vi "GetAllControlReferences.vi"(8 "error in (no error)":errorcluster, 10 "list tab?":bool=TRUE, 11 "VI Refnum in":refnum<vi>) -> (0 "error out":errorcluster, 2 "Ctrl Refs out":refnum<vi>[](array[refnum]), 3 "VI Refnum out":refnum<vi>)   [LabVIEW 2017]
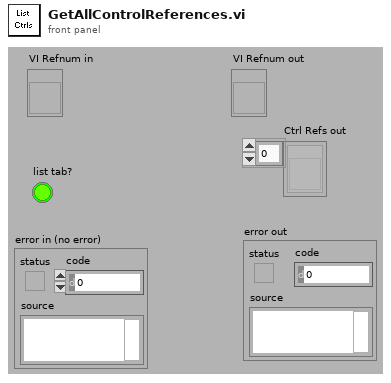
[diagram p1: front panel]
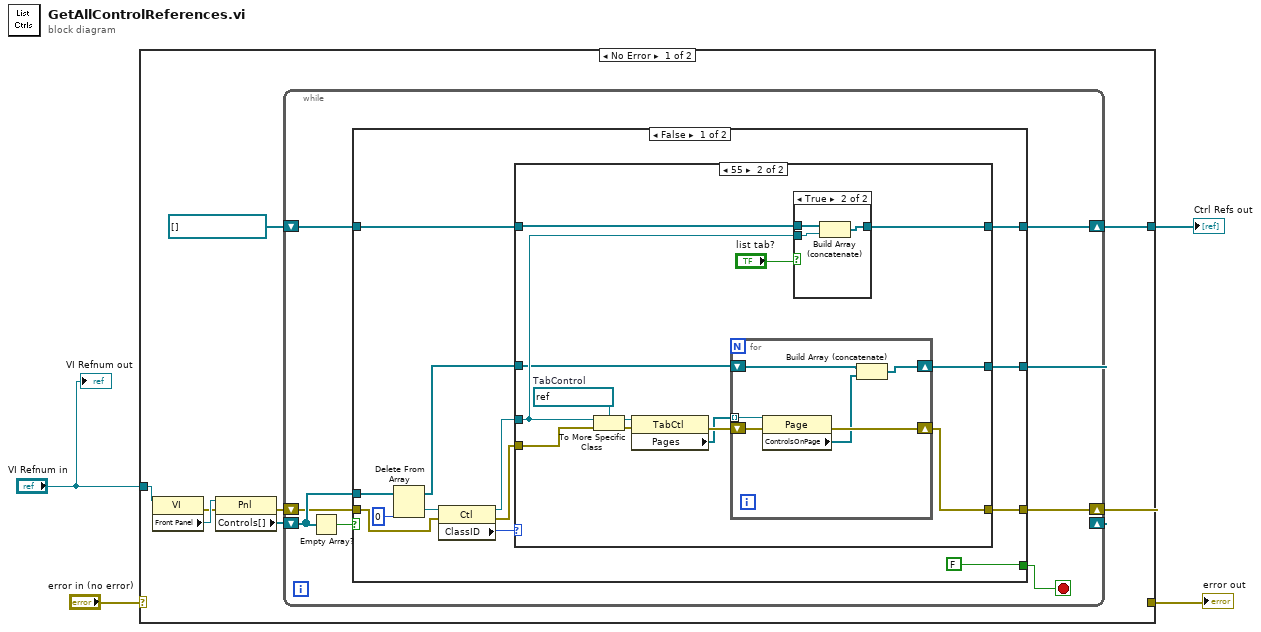
[diagram p0: block diagram]
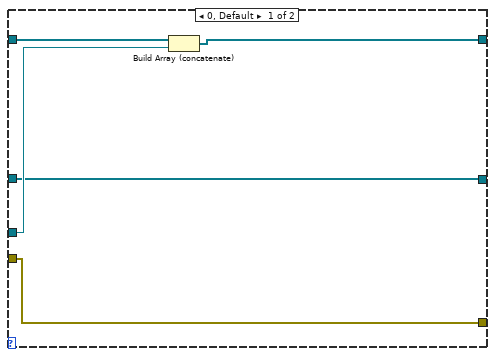
[diagram p2: hidden frame]
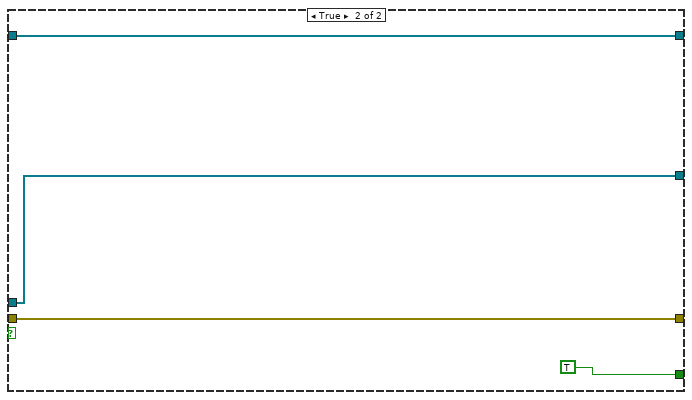
[diagram p4: hidden frame]
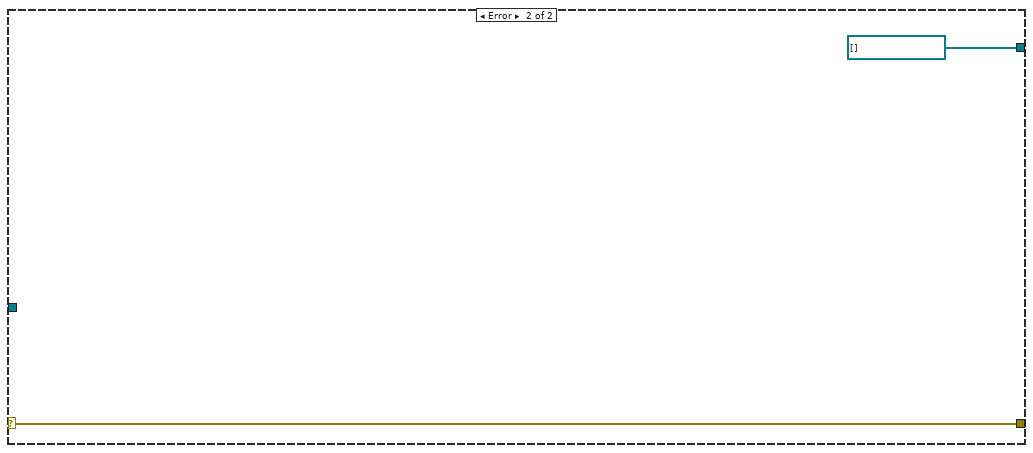
[diagram p5: hidden frame]
diagram:
  n1 = case shown="No Error" "error in (no error)" {
    selector: "error in (no error)" -> [_ w67]
    tunnel: [w6 w67] -> w3
    tunnel: "VI Refnum in" -> [w5 _]
    tunnel: [w8 refnum<vi>[] []] -> w1
    frame No Error {
      n2 = property class="VI"(reference=w5) -> (error out=w11:errorcluster, "Front Panel"=w12:refnum<vi>)  [unwired: 1 in, 1 out]
      n3 = property class="Pnl"(reference=w12, error in=w11) -> (error out=w9:errorcluster, "Controls[]"=w10:refnum<vi>[])  [unwired: 1 out]
      n4 = while {
        shift-right: [w17] -> _
        shift-left: w10 -> [w18]
        shift-right: [w13] -> w6
        shift-left: w9 -> [w16]
        shift-right: [w14] -> w8
        shift-left: refnum<vi>[] [] -> [w15]
        stop <- w19 stop-if-true
        n5 = Empty Array?(array=w18) -> (empty?=w20:bool)
        n6 = case shown="False" w20 {
          tunnel: [FALSE TRUE] -> w19
          tunnel: w18 -> [w31 w65]
          tunnel: [w21 w65] -> w17
          tunnel: w16 -> [w29 w62]
          tunnel: w15 -> [w26 w64]
          tunnel: [w25 w64] -> w14
          tunnel: [w23 w62] -> w13
          frame False {
            n7 = Delete From Array(array=w31, index=0) -> (deleted portion=w30:refnum<vi>, array with subset deleted=w22:refnum<vi>[])  [unwired: 1 in]
            n8 = property class="Ctl"(reference=w30, error in=w29) -> (reference out=w27:refnum<vi>, error out=w24:errorcluster, "ClassID"=w28:u32)
            n9 = case shown="55" w28 {
              tunnel: w27 -> [w37 w43]
              tunnel: w26 -> [w38 w44]
              tunnel: [w36 w41] -> w25
              tunnel: w24 -> [w35 w46]
              tunnel: [w35 w42] -> w23
              tunnel: w22 -> [w34 w40]
              tunnel: [w34 w39] -> w21
              frame 0, Default {
                n10 = Build Array (concatenate)(w38, w37) -> (w36:refnum<vi>[])
              }
              frame 55 {
                w47 = refnum<vi> refnum  # TabControl
                n11 = To More Specific Class(target class=w47, reference=w43, error in=w46) -> (specific class reference=w48:refnum<vi>, error out=w49:errorcluster)
                n12 = property class="TabCtl"(reference=w48, error in=w49) -> (error out=w51:errorcluster, "Pages"=w50:refnum<vi>[])  [unwired: 1 out]
                n13 = for {
                  tunnel: w50 -> [w61] mode=indexing
                  shift-right: [w59] -> w42
                  shift-left: w51 -> [w60]
                  shift-right: [w56] -> w39
                  shift-left: w40 -> [w58]
                  n14 = property class="Page"(reference=w61, error in=w60) -> (error out=w59:errorcluster, "ControlsOnPage"=w57:refnum<vi>[])  [unwired: 1 out]
                  n15 = Build Array (concatenate)(w58, w57) -> (w56:refnum<vi>[])
                }
                n16 = case shown="True" "list tab?" {
                  tunnel: w44 -> [w52 w55]
                  tunnel: w43 -> [_ w54]
                  tunnel: [w52 w53] -> w41
                  frame False {
                  }
                  frame True {
                    n17 = Build Array (concatenate)(w55, w54) -> (w53:refnum<vi>[])
                  }
                }
              }
            }
          }
          frame True {
          }
        }
      }
    }
    frame Error {
    }
  }
  "error out" <- w3
  "Ctrl Refs out" <- w1
  "VI Refnum out" <- "VI Refnum in"
